vi "bind DBL.vi"(8 "error in (no error)":errorcluster, 10 "DBL":dbl, 11 "SQLite3LV Cursor in":refnum<class "cursor.lvclass">) -> (0 "error out":errorcluster, 3 "SQLite3LV Cursor out":refnum<class "cursor.lvclass">)   [LabVIEW 2014, in "SQLite3LV.lvlib" / "cursor.lvclass"]
uses:
  cursor.lvclass
  cursor.lvclass/cursor.ctl
  SQLite3LV.lvlib
  sqlite3_64.dll
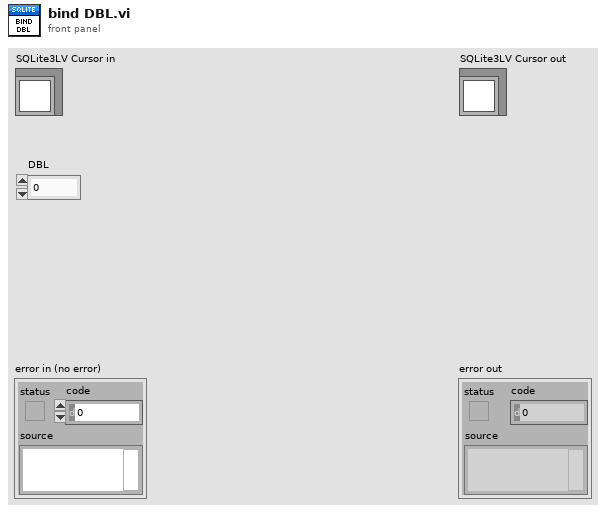
[diagram p1: front panel]
types:
  T1 = typedef "SQLite3LV.lvlib/cursor.lvclass/ctl_active_statement.ctl" = cluster{"ppStmt":i64, "column count":i32, "bind offset":i32, "bind param count":i32, "finished?":bool, "column offset":i32, "column types":i32[]}
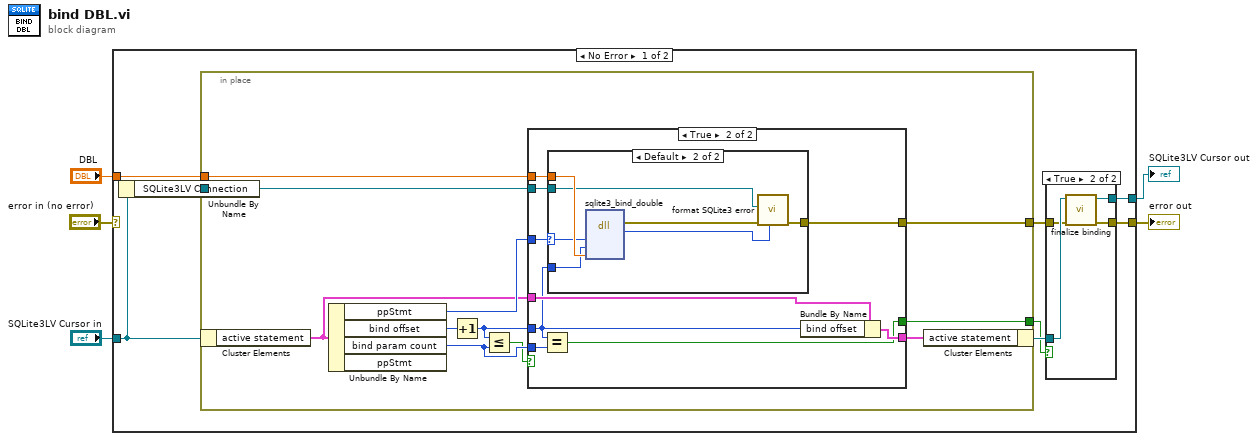
[diagram p0: block diagram]
diagram:
  n1 = case shown="No Error" "error in (no error)" {
    selector: "error in (no error)" -> [_ w49]
    tunnel: [w9 w49] -> w4
    tunnel: [w11 w48] -> w5
    tunnel: "SQLite3LV Cursor in" -> [w8 w48]
    tunnel: "DBL" -> [w13 _]
    frame No Error {
      n2 = Unbundle By Name(w8) -> ("SQLite3LV Connection"=w7:refnum<class "sqlite3.lvclass">)
      n3 = in-place {
        in-place-border: w13 -> [w30]
        in-place-border: [w29] -> w10
        in-place-border: w7 -> [w21]
        in-place-border: [w20] -> w6
        n4 = in-place-cluster #1(w8) -> ("active statement"=w23:T1)
        n5 = Unbundle By Name(w23) -> ("ppStmt"=w28:i64, "bind offset"=w27:i32, "bind param count"=w25:i32)  [unwired: 1 out]
        n6 = Increment(x=w27) -> (x+1=w26:i32)
        n7 = Less Or Equal?(x=w26, y=w25) -> (x <= y?=w24:bool)
        n8 = case shown="True" w24 {
          tunnel: w23 -> [w31 w40]
          tunnel: w30 -> [_ w36]
          tunnel: [w31 w39] -> w22
          tunnel: [_ w38] -> w29
          tunnel: w28 -> [_ w37]
          tunnel: w26 -> [_ w34]
          tunnel: w25 -> [_ w33]
          tunnel: w21 -> [_ w35]
          tunnel: [_ w32] -> w20
          frame False {
          }
          frame True {
            n9 = Equal?(x=w34, y=w33) -> (x = y?=w32:bool)
            n10 = case shown="Default" w37 {
              selector: w37 -> [_ w44]
              tunnel: [_ w47] -> w38
              tunnel: w34 -> [_ w43]
              tunnel: w36 -> [_ w45]
              tunnel: w35 -> [_ w42]
              frame 0 {
              }
              frame Default {
                n11 = dll-call lib="C:/Users/BobUser/Desktop/LVTables/sqlite3**.*" fn="sqlite3_bind_double"("pStmt"=w44, "index"=w43, "value"=w45) -> (error out=w46:errorcluster, "column count"=w41:i32)  [unwired: 6 in, 1 out]
                n12 = call "format SQLite3 error.vi"("SQLite3LV Connection result"=w41, "error in (no error)"=w46, "psqlite"=w42) -> ("error out"=w47:errorcluster)  [unwired: 8 in]
              }
            }
            n13 = Bundle By Name(cluster=w40, "bind offset"=w34) -> (w39:T1)
          }
        }
        n14 = in-place-cluster #1("active statement"=w22) -> (w12:refnum<class "cursor.lvclass">)
      }
      n15 = case shown="True" w6 {
        tunnel: w12 -> [w15 w19]
        tunnel: [w15 w18] -> w11
        tunnel: w10 -> [w14 w17]
        tunnel: [w14 w16] -> w9
        frame False {
        }
        frame True {
          n16 = call "finalize binding.vi"("error in (no error)"=w17, "SQLite3LV Cursor in"=w19) -> ("error out"=w16:errorcluster, "SQLite3LV Cursor out"=w18:refnum<class "cursor.lvclass">)  [unwired: 8 in]
        }
      }
    }
    frame Error {
    }
  }
  "error out" <- w4
  "SQLite3LV Cursor out" <- w5
